vi "InitDAQ.vi"(3 "error in":errorcluster) -> (0 "error out":errorcluster, 2 "DAQ connected?":bool)   [LabVIEW 2013]
uses:
  <vilib>/DAQmx/create/channels.llb/DAQmx Create Channel (AI-Voltage-Basic).vi
  <vilib>/DAQmx/configure/timing.llb/DAQmx Timing (Sample Clock).vi
panel:
  out "task out":refnum<k21>
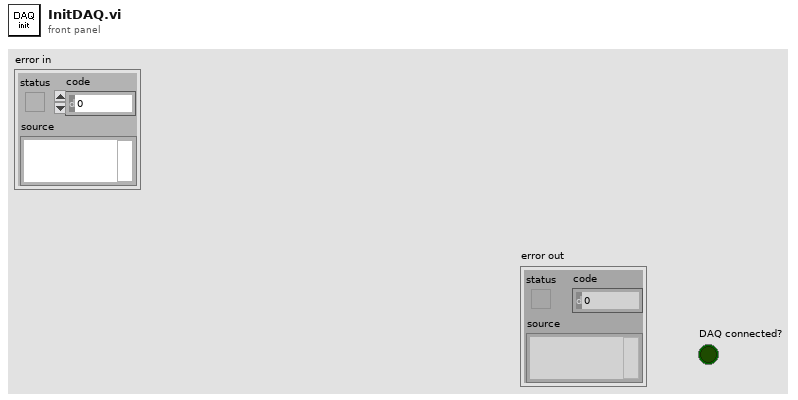
[diagram p1: front panel]
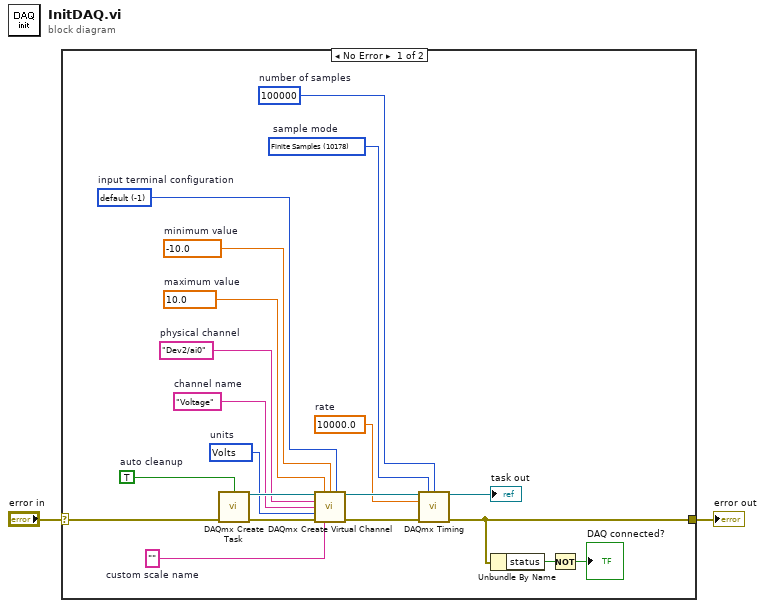
[diagram p0: block diagram]
diagram:
  n1 = case shown="No Error" "error in" {
    selector: "error in" -> [w3 w23]
    tunnel: [w4 w23] -> w1
    frame No Error {
      w7 = 10178 items=["Finite Samples"=10178, "Continuous Samples"=10123, "Hardware Timed Single Point"=12522]  # sample mode
      w8 = 100000  # number of samples
      w9 = 10000.0  # rate
      w12 = -1 items=["default"=-1, "RSE"=10083, "NRSE"=10078, "Differential"=10106, "Pseudodifferential"=12529]  # input terminal configuration
      w13 = 10348 items=["Volts"=10348, "From Custom Scale"=10065]  # units
      w14 = "Voltage"  # channel name
      w16 = ""  # custom scale name
      w17 = -10.0  # minimum value
      w18 = 10.0  # maximum value
      w19 = "Dev2/ai0"  # physical channel
      w21 = TRUE  # auto cleanup
      n2 = call <vilib>:"DAQmx Create Task.vi"("auto cleanup"=w21, "error in"=w3) -> ("task out"=w20:refnum<k21>, "error out"=w22:errorcluster)  [unwired: 12 in]
      n3 = call-poly <vilib>:"DAQmx Create Virtual Channel.vi"("task in"=w20, "maximum value"=w18, "minimum value"=w17, "input terminal configuration"=w12, "physical channels"=w19, "name to assign"=w14, "units"=w13, "error in"=w22, "custom scale name"=w16) -> ("task out"=w10:refnum<k21>, "error out"=w15:errorcluster)  [unwired: 5 in]
      n4 = call-poly <vilib>:"DAQmx Timing.vi"("task/channels in"=w10, "sample mode"=w7, "samples per channel"=w8, "rate"=w9, "error in"=w15) -> ("task out"=→"task out":refnum<k21>, "error out"=w4:errorcluster)  [unwired: 9 in]
      n5 = Unbundle By Name(w4) -> ("status"=w6:bool)
      n6 = Not(x=w6) -> (.not. x?=→"DAQ connected?":bool)
    }
    frame Error {
    }
  }
  "error out" <- w1
